vi "Write alpha_n0.vi"(8 "error in (no error)":errorcluster, 10 "alpha_n0":dbl, 11 "Analytical Serial Arm Class in":refnum<class "NI_Robotics_Analytical Serial Arm Class.lvclass">) -> (0 "error out":errorcluster, 3 "Analytical Serial Arm Class out":refnum<class "NI_Robotics_Analytical Serial Arm Class.lvclass">)   [LabVIEW 2017, in "NI_Robotics_Analytical Serial Arm Class.lvclass"]
uses:
  <vilib>/robotics/Kinematics/Analytical/Generic/NI_Robotics_Analytical Serial Arm Class.lvclass
  <vilib>/robotics/Kinematics/Analytical/Generic/NI_Robotics_Analytical Serial Arm Class.lvclass/NI_Robotics_Analytical Serial Arm Class.ctl
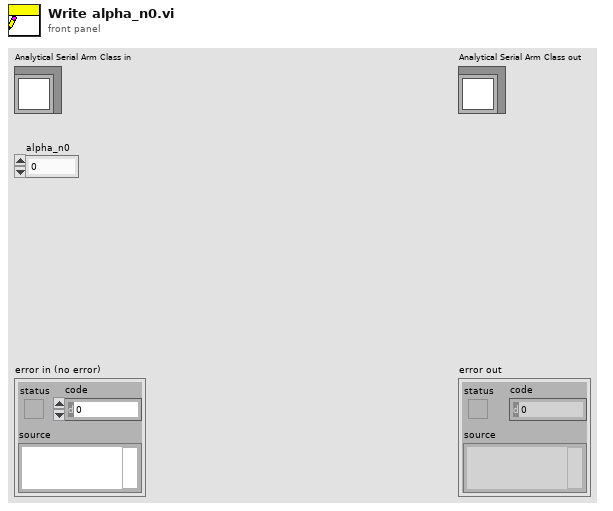
[diagram p1: front panel]
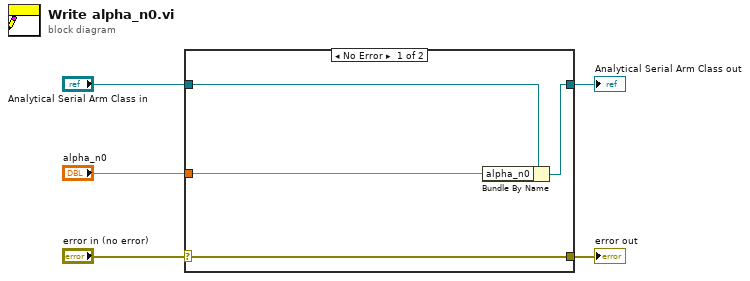
[diagram p0: block diagram]
diagram:
  n1 = case shown="No Error" "error in (no error)" {
    selector: "error in (no error)" -> [w9 w10]
    tunnel: [w9 w10] -> w4
    tunnel: [w7 w11] -> w2
    tunnel: "Analytical Serial Arm Class in" -> [w8 w11]
    tunnel: "alpha_n0" -> [w6 _]
    frame No Error {
      n2 = Bundle By Name(cluster=w8, "alpha_n0"=w6) -> (w7:refnum<class "NI_Robotics_Analytical Serial Arm Class.lvclass">)
    }
    frame Error {
    }
  }
  "error out" <- w4
  "Analytical Serial Arm Class out" <- w2
